vi "I16_Static Read.vi"(8 "error in (no error)":errorcluster, 9 "Default":i16, 11 "Tag Name":string) -> (0 "error out":errorcluster, 1 "Value":i16)   [LabVIEW 2010, in "Current Value Table.lvlib"]
doc: "This VI will read the data associated with a single tag. This VI will only look up the tag index on the first call, or if the look-up resulted in an error. This VI has higher performance than the normal read function thanks to the removal of the name check."
uses:
  Current Value Table.lvlib
  Type Defs/Memory Commands.ctl
  FGVs/Tag Memory Methods.ctl
  I16_Memory Block.vi
  I16_Type To Enum.vi
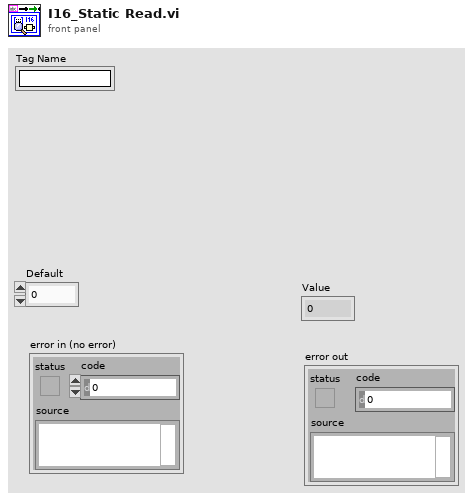
[diagram p1: front panel]
types:
  T1 = typedef "Current Value Table.lvlib/Tag Memory Methods.ctl" = enum16{"Clear", "Read Tag Index", "Read Tag Indices", "Generate Group", "Add Tag", "Overwrite Tag", "Read Description", "Get Stored Tags"}
  T2 = typedef "Current Value Table.lvlib/Data Types.ctl" = enum16{"Double", "Single", "I64", "I32", "I16", "I8", "U64", "U32", "U16", "U8", "String", "Boolean", "Array of U8", "Array of U16", "Array of U32", "Array of U64", "Array of I64", "Array of I32", "Array of I16", "Array of I8", "Array of Double", "Array of Single", "Array of Boolean", "Array of String"}
  T3 = typedef "Current Value Table.lvlib/Memory Commands.ctl" = enum16{"Init", "Add Data", "Read", "Read Group", "Read All", "Write", "Write Group", "Get Size"}
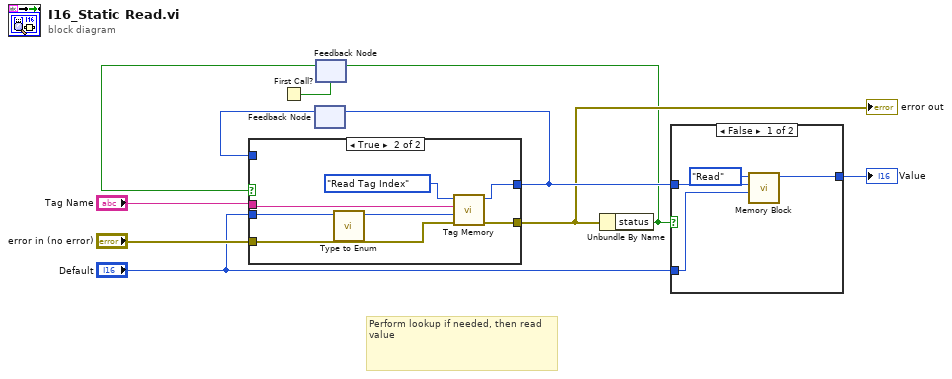
[diagram p0: block diagram]
diagram:
  # "Perform lookup if needed, then read value"
  n1 = First Call?() -> (First Call?: T/F=w3:bool)
  n2 = feedback #1() -> (w9:i32)  [unwired: 1 in]
  n3 = feedback #2(w3) -> (w2:bool)
  n4 = case shown="True" w2 {
    tunnel: [w12 w17] -> w6
    tunnel: "error in (no error)" -> [w12 w16]
    tunnel: [w11 w14] -> w8
    tunnel: w9 -> [w11 _]
    tunnel: "Tag Name" -> [_ w15]
    tunnel: "Default" -> [_ w13]
    frame False {
    }
    frame True {
      n5 = call-poly "Type to Enum.vi"("Default"=w13) -> ("Data Type Enum"=w19:T2)  [unwired: 10 in]
      n6 = call "Tag Memory.vi"("error in (no error)"=w16, "Expected Type"=w19, "Tag"=w15, "Method"=Tag_Memory_Methods."Read Tag Index") -> ("error out"=w17:errorcluster, "Index Out"=w14:i32)  [unwired: 2 in, 4 out]
    }
  }
  "error out" <- w6
  n7 = feedback-in #1(w8) -> ()
  n8 = Unbundle By Name(w6) -> ("status"=w5:bool)
  n9 = feedback-in #2(w5) -> ()
  n10 = case shown="False" w5 {
    tunnel: w8 -> [w22 _]
    tunnel: "Default" -> [w21 w24]
    tunnel: [w20 w24] -> w4
    frame False {
      n11 = call-poly "Memory Block.vi"("Value"=w21, "Index"=w22, "Method"=Memory_Commands."Read") -> ("Value Out"=w20:i16)  [unwired: 6 in, 2 out]
    }
    frame True {
    }
  }
  "Value" <- w4
